vi "callMatlab.vi"() -> ()   [LabVIEW 2011, in "run.lvlib"]
uses:
  run.lvlib
panel:
  out "String":string
  out "Path":path
  out "error out":errorcluster
  out "Real":dbl
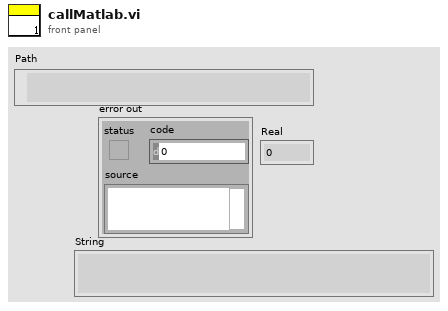
[diagram p1: front panel]
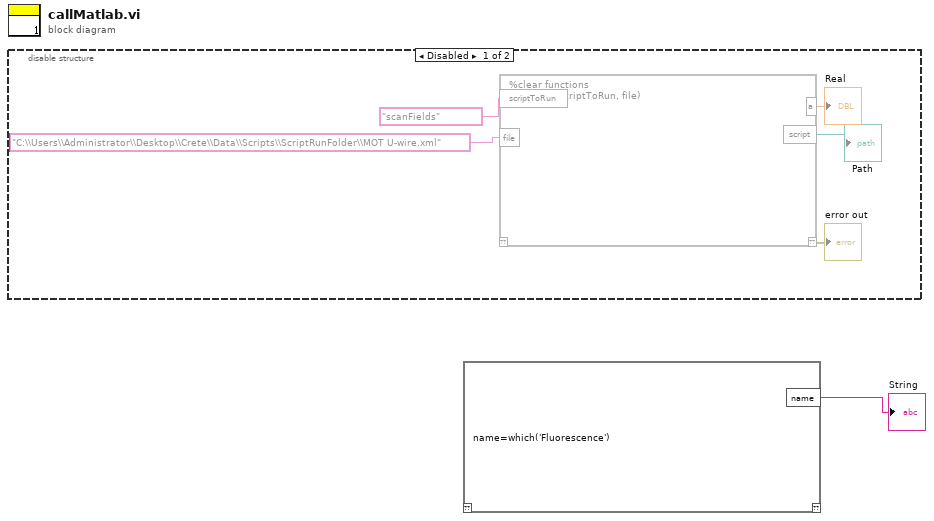
[diagram p0: block diagram]
diagram:
  n1 = disable-structure shown="Disabled" {
    frame Disabled {
      n2 = script code="%clear functions\n%a=feval(scriptToRun, file)"("scriptToRun"="scanFields", "file"="C:\\Users\\Administrator\\Desktop\\Crete\\Data\\Scripts\\ScriptRunFolder\\MOT U-wire.xml") -> ("??"=→"error out":errorcluster, "a"=→"Real":dbl, "script"=→"Path":path)  [unwired: 1 in]
    }
    frame Enabled {
    }
  }
  n3 = script code="name=which('Fluorescence')"() -> ("name"=→"String":string)  [unwired: 1 in, 1 out]
